vi "O_Data_to_Excel.vi"(8 "error in (no error)":errorcluster, 9 "ALL RESULT Array":dbl[][](array[numeric]) format="%_9g", 10 "REQUEST #":string, 11 "PROJECT #":string) -> (0 "error out":errorcluster)   [LabVIEW 2020]
uses:
  <vilib>/Utility/NIReport.llb/Report Type.ctl
  <vilib>/addons/_office/excel.llb/Excel Easy Table (num).vi
  <vilib>/Utility/NIReport.llb/NI_report.lvclass
  <vilib>/addons/_office/NI_ReportGenerationToolkit.lvlib
  <vilib>/Utility/NIReport.llb/Excel/NI_Excel.lvclass
  <vilib>/Utility/NIReport.llb/NI_ReportGenerationCore.lvlib
panel:
  # "Column 7"
  # "Column 8"
  # "Column 9"
  # "Column 10"
  # "Column 11"
  # "Column 12"
  # "Column 13"
  # "Column 14"
  # "Column 15"
  # "Column 2"
  # "Column 3"
  # "Column 4"
  # "Column 5"
  # "Column 6"
  # "Column 0"
  # "Column 1"
  # "Ta\n(ns)"
  # "Tb\n(ns)"
  # "Trr\n(ns)"
  # "Irrm\n(A)"
  # "Qrr\n(nC)"
  # "Erec\n(uJ)"
  # "Di/Dt\n(A/us)"
  # "Di\n(A)"
  # "Dt\n(us)"
  # "Vce"
  # "Ice"
  # "Vge"
  # "Rg"
  # "Temperature"
  # "DUT  #"
  # "TEST #"
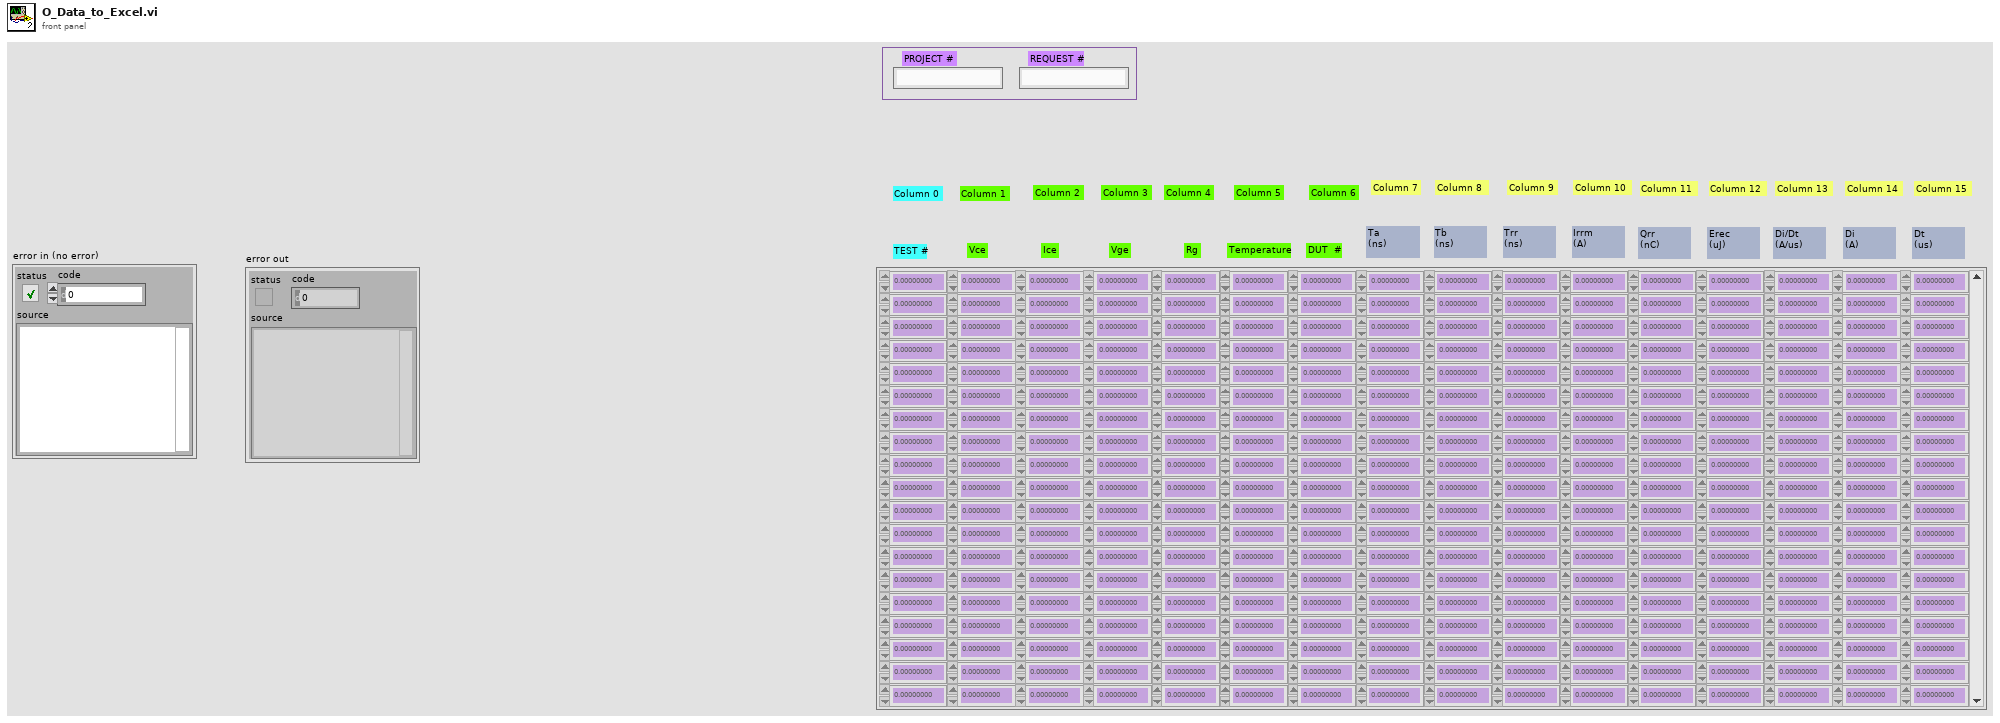
[diagram p1: front panel]
types:
  T1 = typedef "NI_ReportGenerationCore.lvlib/Report Type.ctl" = enum16{"HTML", "Word", "Excel"}
  T2 = enum16{"maximized", "minimized", "normal", "no change"}
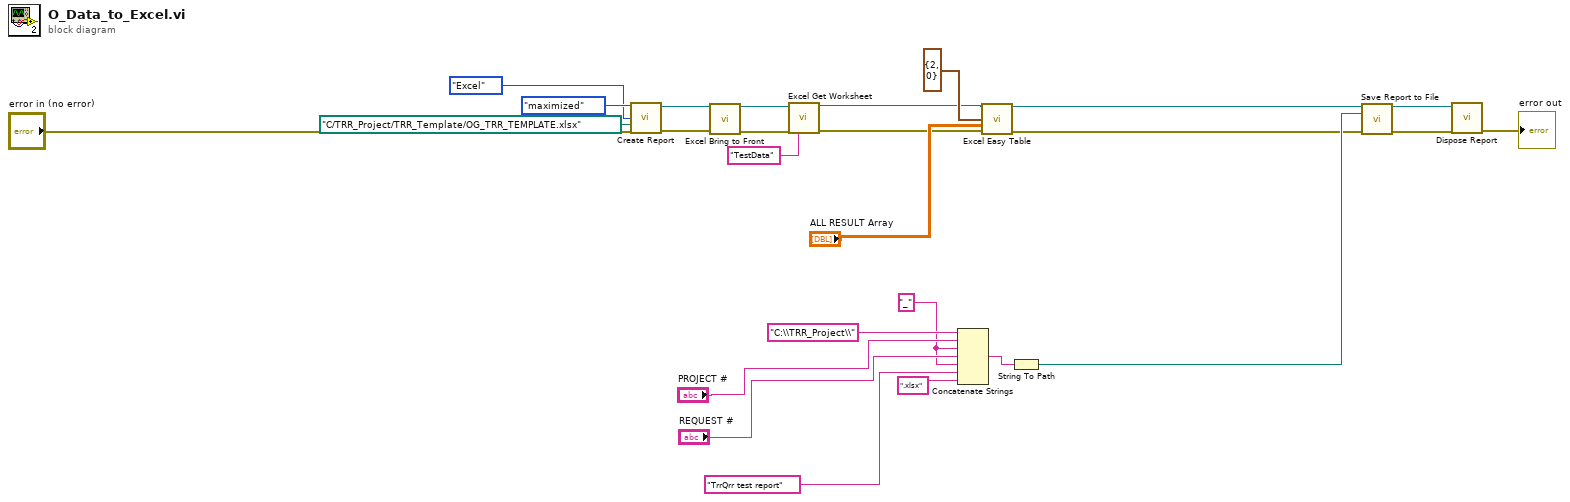
[diagram p0: block diagram]
diagram:
  w8 = "_" ("string")
  n1 = call <vilib>:"Create Report.vi"("window state (normal)"=T2."maximized", "report type"=Report_Type."Excel", "template (empty)"=path "C:/TRR_Project/TRR_Template/OG_TRR_TEMPLATE.xlsx", "error in (no error)"="error in (no error)") -> ("report out"=w4:refnum<class "NI_report.lvclass">, "error out"=w6:errorcluster)  [unwired: 10 in]
  n2 = call <vilib>:"Excel Bring to Front.vi"("report in"=w4, "error in (no error)"=w6) -> ("report out"=w3:refnum<class "NI_report.lvclass">, "error out"=w5:errorcluster)  [unwired: 12 in]
  n3 = call <vilib>:"Excel Get Worksheet.vi"("report in"=w3, "error in (no error)"=w5, "name (\"\")"="TestData" ("name (\"\")")) -> ("report out"=w15:refnum<class "NI_report.lvclass">, "error out"=w16:errorcluster)  [unwired: 11 in]
  n4 = Concatenate Strings("C:\\TRR_Project\\" ("string"), "PROJECT #", w8, "REQUEST #", w8, "TrrQrr test report" ("string"), ".xlsx" ("string")) -> (w26:string)
  n5 = call-poly <vilib>:"Excel Easy Table.vi"("report in"=w15, "start (0, 0)"=cluster{"row":i32, "column":i32} {"row"=2, "column"=0}, "text data"="ALL RESULT Array", "error in (no error)"=w16) -> ("report out"=w1:refnum<class "NI_report.lvclass">, "error out"=w2:errorcluster)  [unwired: 7 in, 3 out]
  n6 = String To Path(string=w26) -> (path=w14:path)
  n7 = call-dynamic "Save Report to File.vi"("report in"=w1, "report file path"=w14, "error in (no error)"=w2) -> ("report out"=w12:refnum<class "NI_report.lvclass">, "error out"=w13:errorcluster)  [unwired: 11 in]
  n8 = call-dynamic "Dispose Report.vi"("report in"=w12, "error in (no error)"=w13) -> ("error out"=→"error out":errorcluster)  [unwired: 13 in]
